vi "Write to CSV.vi"(0 "Path In":path, 5 "Array In":string[][](array[string]), 7 "Append to File?":bool, 11 "Error In":errorcluster) -> (4 "Path Out":path, 6 "Log Data":string, 15 "Error Out":errorcluster)   [LabVIEW 2023, in "File and Path Operations.lvlib"]
doc: "This VI writes a string array to a CSV file, with each array element on a new line."
uses:
  File and Path Operations.lvlib
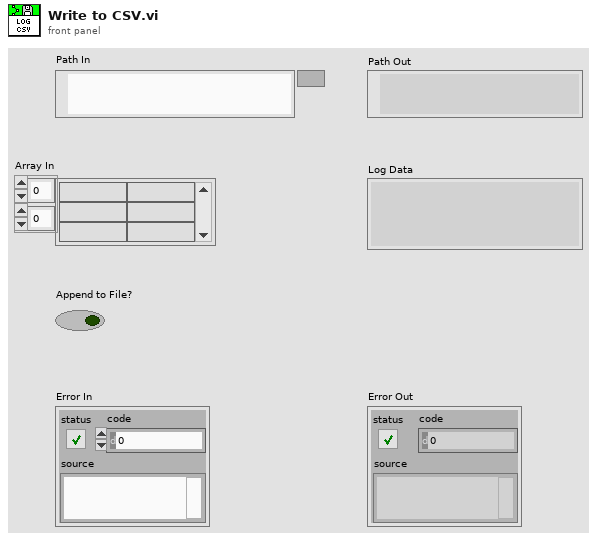
[diagram p1: front panel]
types:
  T1 = enum16{"open", "replace", "create", "open or create", "replace or create", "replace or create with confirmation"}
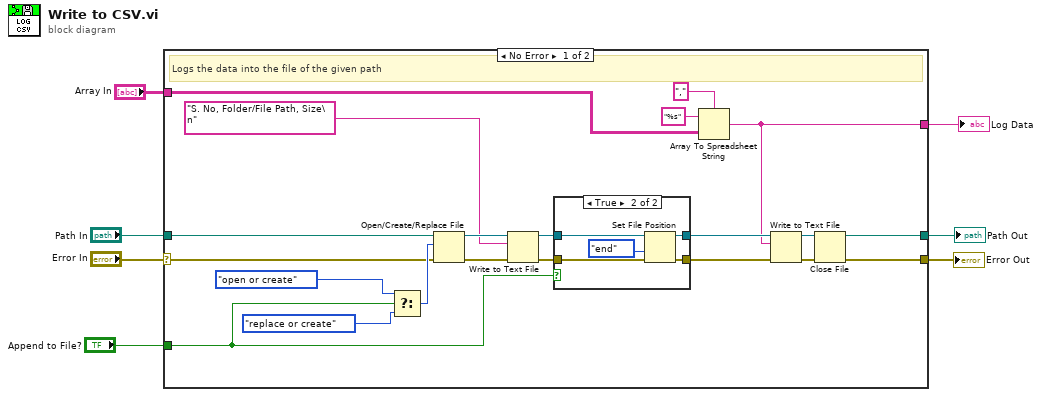
[diagram p0: block diagram]
diagram:
  n1 = case shown="No Error" "Error In" {
    selector: "Error In" -> [w20 w36]
    tunnel: [w25 w36] -> w6
    tunnel: "Path In" -> [w12 _]
    tunnel: "Append to File?" -> [w11 _]
    tunnel: [w10 _] -> w2
    tunnel: "Array In" -> [w9 _]
    tunnel: [w8 _] -> w1
    frame No Error {
      # "Logs the data into the file of the given path"
      n2 = Select ("function")(t=T1."open or create" ("operation (0:open)"), s=w11, f=T1."replace or create" ("operation (0:open)")) -> (s? t:f=w21:T1)
      n3 = Open/Create/Replace File(file path (use dialog)=w12, error in=w20, operation (0:open)=w21) -> (refnum out=w15:refnum<file>, error out=w14:errorcluster)  [unwired: 3 in, 1 out]
      n4 = Write to Text File(file (use dialog)=w15, text="S. No, Folder/File Path, Size\n", error in=w14) -> (refnum out=w17:refnum<file>, error out=w16:errorcluster)  [unwired: 1 in, 1 out]
      n5 = case shown="True" w11 {
        tunnel: w16 -> [w29 w35]
        tunnel: [w29 w34] -> w19
        tunnel: w17 -> [w30 w32]
        tunnel: [w30 w33] -> w18
        frame False {
        }
        frame True {
          n6 = Set File Position(refnum=w32, from (0:start)=enum16{"start", "end", "current"}."end", error in=w35) -> (refnum out=w33:refnum<file>, error out=w34:errorcluster)  [unwired: 1 in]
        }
      }
      n7 = Array To Spreadsheet String(delimiter (Tab)=",", array=w9, 3:"%s" ("format string")) -> (spreadsheet string=w8:string)
      n8 = Write to Text File(file (use dialog)=w18, text=w8, error in=w19) -> (refnum out=w27:refnum<file>, error out=w26:errorcluster)  [unwired: 1 in, 1 out]
      n9 = Close File(refnum=w27, error in=w26) -> (path=w10:path, error out=w25:errorcluster)
    }
    frame Error {
    }
  }
  "Error Out" <- w6
  "Path Out" <- w2
  "Log Data" <- w1
